vi "GetDriverName.vi"(8 "Error In":errorcluster, 11 "reference in":refnum<class "VdDigitalControl_DAQmx.lvclass">) -> (0 "Error Out":errorcluster, 2 "DriverName":string, 3 "reference in":refnum<class "VdDigitalControl_DAQmx.lvclass">)   [LabVIEW 2020, in "VdDigitalControl_DAQmx.lvclass"]
uses:
  VdDigitalControl_DAQmx.lvclass
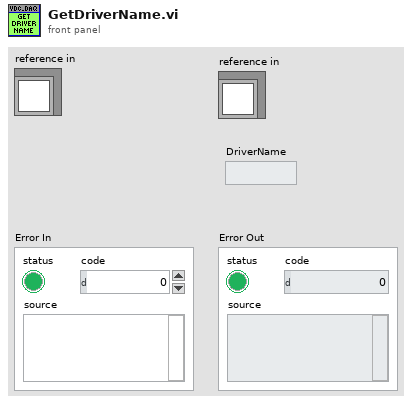
[diagram p1: front panel]
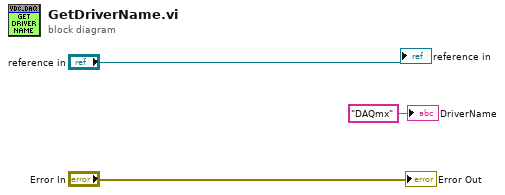
[diagram p0: block diagram]
diagram:
  "Error Out" <- "Error In"
  "reference in" <- "reference in"
  "DriverName" <- "DAQmx" ("DriverName")
